vi "DecodeBallReplacement.vi"(1 "element":u8[](array[numeric]), 5 "error in (no error)":errorcluster) -> (14 "BallReplacement":cluster{"x":dbl, "y":dbl, "vx":dbl, "vy":dbl}, 15 "element 2":u8[](array[numeric]), 19 "error out":errorcluster)   [LabVIEW 2023, in "Referee.lvclass"]
uses:
  Referee.lvclass
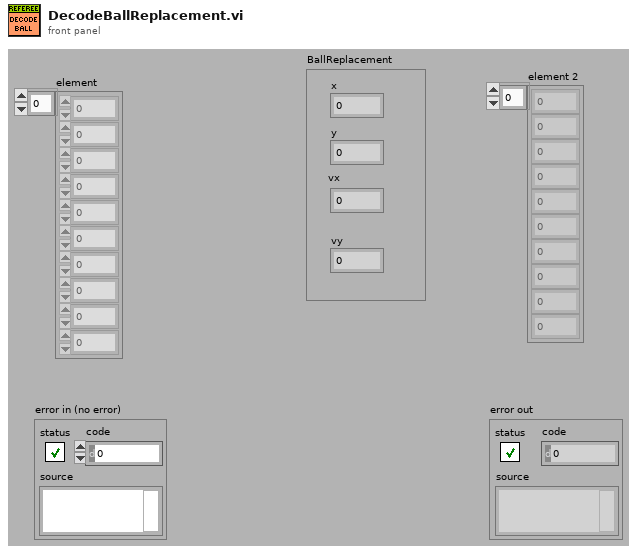
[diagram p1: front panel]
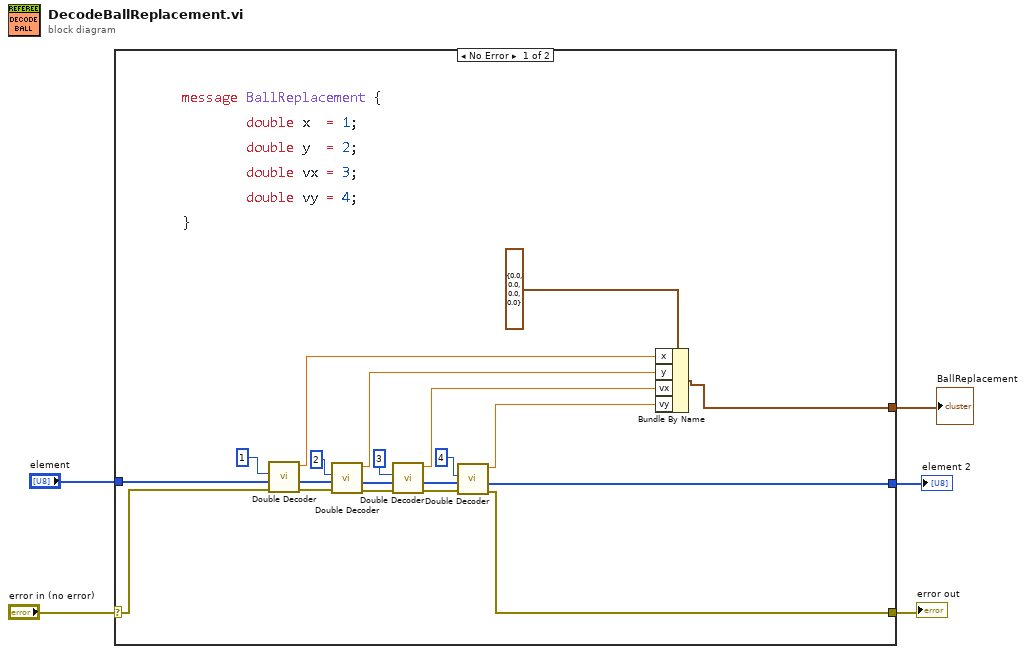
[diagram p0: block diagram]
diagram:
  n1 = case shown="No Error" "error in (no error)" {
    selector: "error in (no error)" -> [w23 w26]
    tunnel: [w13 w26] -> w4
    tunnel: "element" -> [w25 _]
    tunnel: [w12 _] -> w2
    tunnel: [w11 _] -> w1
    frame No Error {
      n2 = call "Double Decoder.vi"("error in (no error)"=w23, "Array"=w25, "Key"=1) -> ("error out"=w20:errorcluster, "array w/ subset deleted"=w18:u8[], "Double"=w10:dbl)  [unwired: 5 in, 1 out]
      n3 = call "Double Decoder.vi"("error in (no error)"=w20, "Array"=w18, "Key"=2) -> ("error out"=w22:errorcluster, "array w/ subset deleted"=w21:u8[], "Double"=w9:dbl)  [unwired: 5 in, 1 out]
      n4 = call "Double Decoder.vi"("error in (no error)"=w22, "Array"=w21, "Key"=3) -> ("error out"=w19:errorcluster, "array w/ subset deleted"=w14:u8[], "Double"=w8:dbl)  [unwired: 5 in, 1 out]
      n5 = call "Double Decoder.vi"("error in (no error)"=w19, "Array"=w14, "Key"=4) -> ("error out"=w13:errorcluster, "array w/ subset deleted"=w12:u8[], "Double"=w7:dbl)  [unwired: 5 in, 1 out]
      n6 = Bundle By Name(cluster=cluster{"x":dbl, "y":dbl, "vx":dbl, "vy":dbl} {"x"=0.0, "y"=0.0, "vx"=0.0, "vy"=0.0} ("BallReplacement 2"), "x"=w10, "y"=w9, "vx"=w8, "vy"=w7) -> (w11:cluster{"x":dbl, "y":dbl, "vx":dbl, "vy":dbl})
    }
    frame Error {
    }
  }
  "error out" <- w4
  "element 2" <- w2
  "BallReplacement" <- w1
